vi "Process.vi"(8 "error in (no error)":errorcluster, 11 "Analyzer":refnum<class "Analyzer.lvclass">) -> (0 "error out":errorcluster, 3 "Analyzer out":refnum<class "Analyzer.lvclass">)   [LabVIEW 2022 SP3, in "Analyzer.lvclass"]
uses:
  Analyzer.lvclass
  C:/Program Files (x86)/National Instruments/LabVIEW 2022/vi.lib/JKI/JKI SMO/SMO/SMO.lvclass
  <vilib>/JKI/JKI SMO/SMO/Typedefs/Parent Call--Enum.ctl
  Typedefs/PublicEvents--Analyzer.NewEventMessage.ctl
  <vilib>/JKI/JKI SMO/SMO/SMO.lvclass
  <vilib>/JKI/JKI SMO/SMO/SMO.lvclass/SMO.ctl
  2a4e98fd-c6f0-4dfa-82c0-cf19db74dbf6.vi
  <vilib>/JKI/JKI SMO/SMO/Private/GetVariant(Attr).vi
  <vilib>/JKI/JKI SMO/Support/Attribute.Identity/Read UniqueName.vi
  <vilib>/JKI/JKI SMO/Support/Attribute.Identity/Read Given Name.vi
  <vilib>/JKI/JKI SMO/Support/Attribute.Identity/Read ProspectiveOwner.vi
  <vilib>/JKI/JKI SMO/SMO/Private/ReftoDVR--SMO.vi
  <vilib>/Utility/file.llb/Write Delimited Spreadsheet (string).vi
  <vilib>/JKI/JKI SMO/Support/Attribute.Identity/Attribute.Identity.lvclass
panel:
  in  "Save":bool
  in  "Word or Phrase:":string
  in  "Search By:":string(combo)
  in  "Start Button":bool
  out "Table Report":string[][](table)
  in  "OK":bool
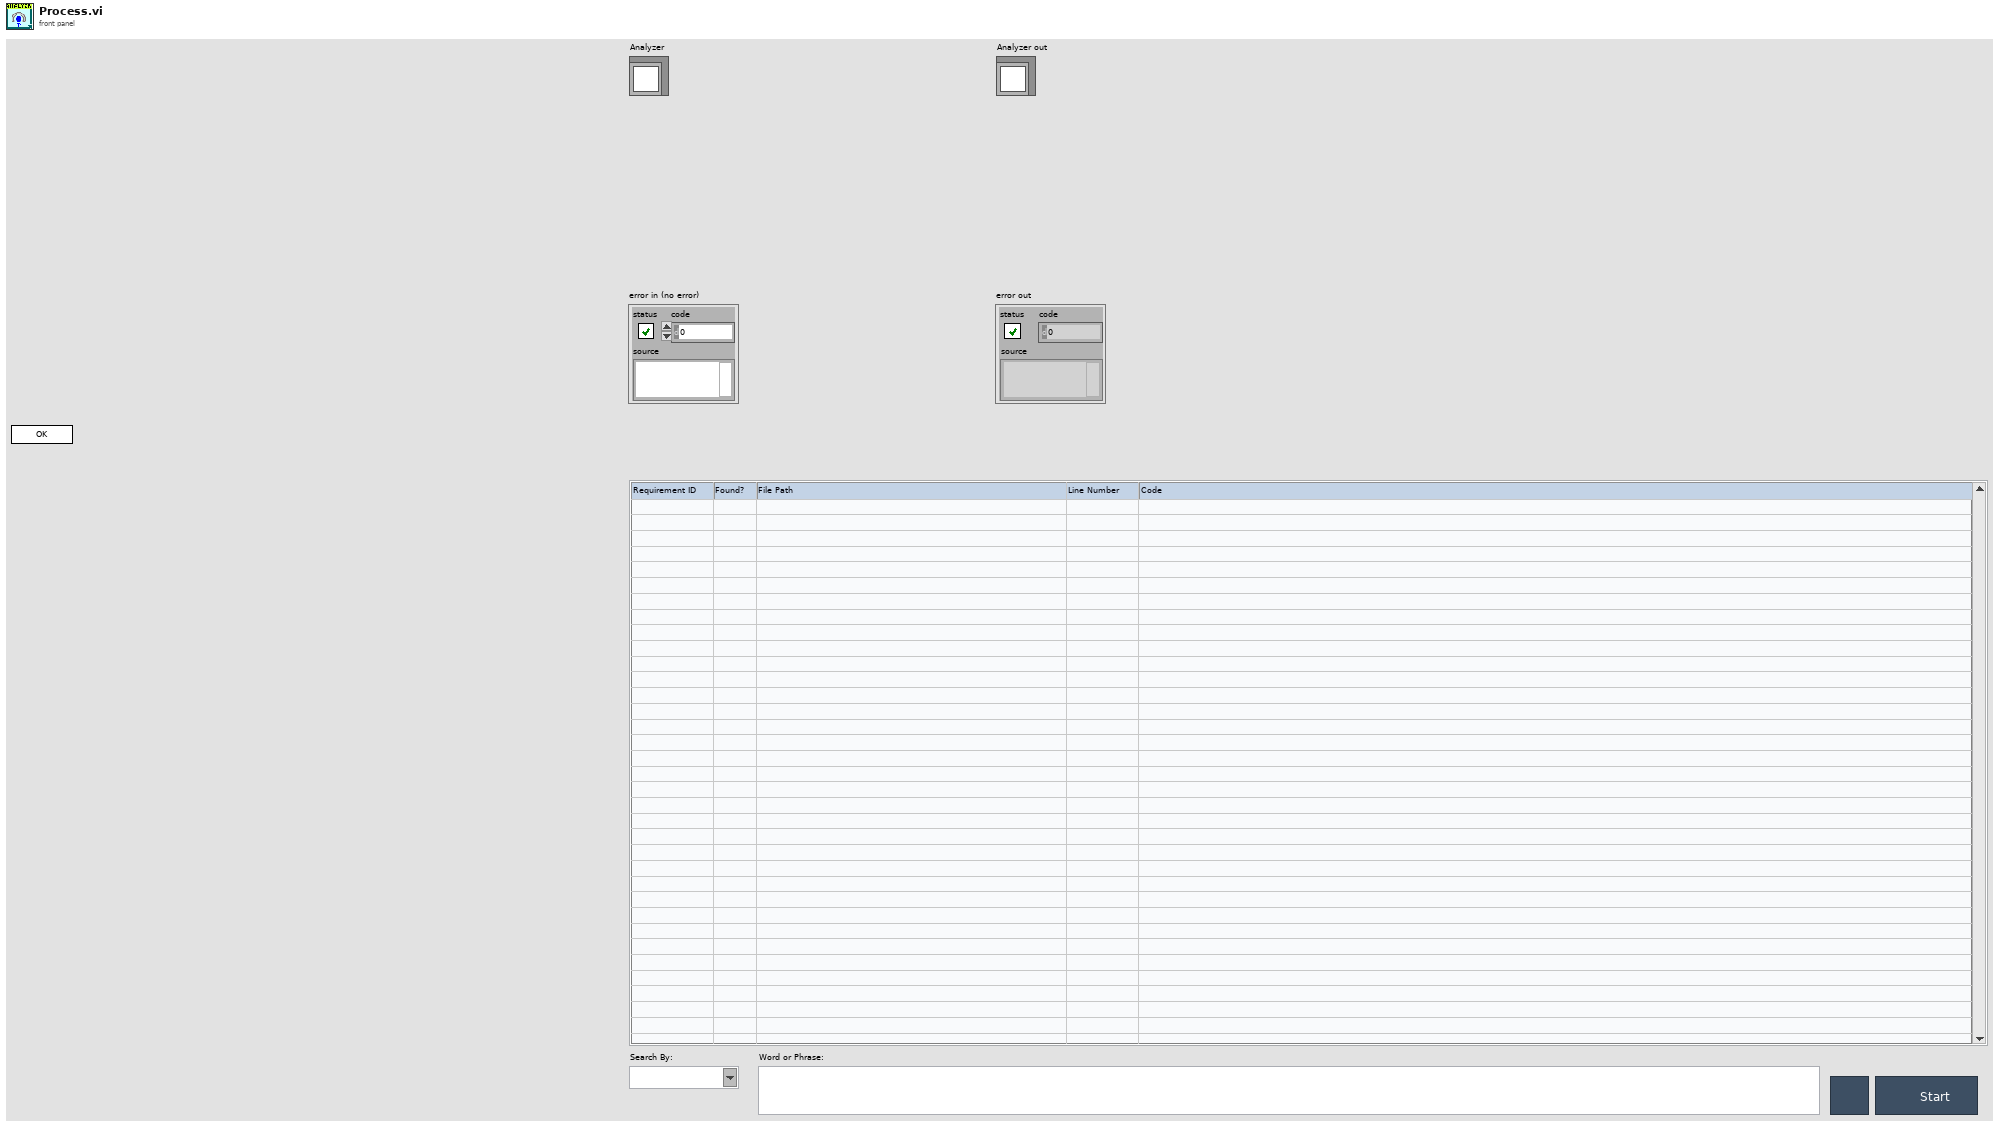
[diagram p1: front panel]
types:
  T1 = typedef "SMO.lvclass/Parent Call--Enum.ctl" = enum16{"Allows parent to run", "Does not request parent to run"}
  T2 = typedef "Analyzer.lvclass/PublicEvents--Analyzer.NewEventMessage.ctl" = cluster{"Title":string, "Message":variant}
  T3 = cluster{"Requirements Directory":path, "Report Generation Save Path":path, "Source Code to Directory":path, "Search By:":string, "Word/Phrase:":string, "Source Code File":path}
  T4 = enum8{"Enabled", "Disabled", "Disabled and Grayed Out"}
  T5 = enum32{"invalid app kind", "Development System", "Run Time System", "Student Edition", "Embedded LabVIEW", "Evaluation", "Custom"}
  T6 = enum32{"Invalid", "Standard", "Closed", "Hidden", "Minimized", "Maximized"}
  T7 = typedef "Analyzer.lvclass/Analyzer State--enum.ctl" = enum16{"unknown", "Opened", "Embedded", "Closed"}
  T8 = cluster{"Requirements Directory":path, "Report Generation Save Path":path, "Source Code Directory":path, "Search By:":string, "Word/Phrase:":string, "Source Code File":path}
  T9 = cluster{"Core":cluster{"Current VI Reference":refnum<vi>, "Close Panel on Exit?":bool, "error":errorcluster}, "Self Ref":refnum<class "Analyzer.lvclass">, "Python":cluster{"Ref":refnum<k35>, "SReTT_script":path}, "Settings":cluster{"Requirements Directory":path, "Report Generation Save Path":path, "Source Code Directory":path, "Search By:":string, "Word/Phrase:":string, "Source Code File":path}, "Table":string[][], "Requirement to Look":string, "Requirements":string[], "Req Files Done":bool, "Code Files Done":bool, "Single Word":bool, "S Word Ctrl":bool}
  T10 = cluster{"Current VI Reference":refnum<vi>, "Close Panel on Exit?":bool, "error":errorcluster}
  T11 = typedef "SMO.lvclass/Protected Events.ctl" = cluster{"StopProcesses":refnum<user-event>, "AbortProcesses":refnum<user-event>, "Config Changed":refnum<user-event>, "Dependency":refnum<user-event>}
  T12 = typedef "Analyzer.lvclass/PublicEvents--Cluster.ctl" = cluster{"UI State":refnum<user-event>, "NewEventMessage":refnum<user-event>}
  T13 = typedef "Analyzer.lvclass/PrivateEvents--Cluster.ctl" = cluster{"NewRequest":refnum<user-event>}
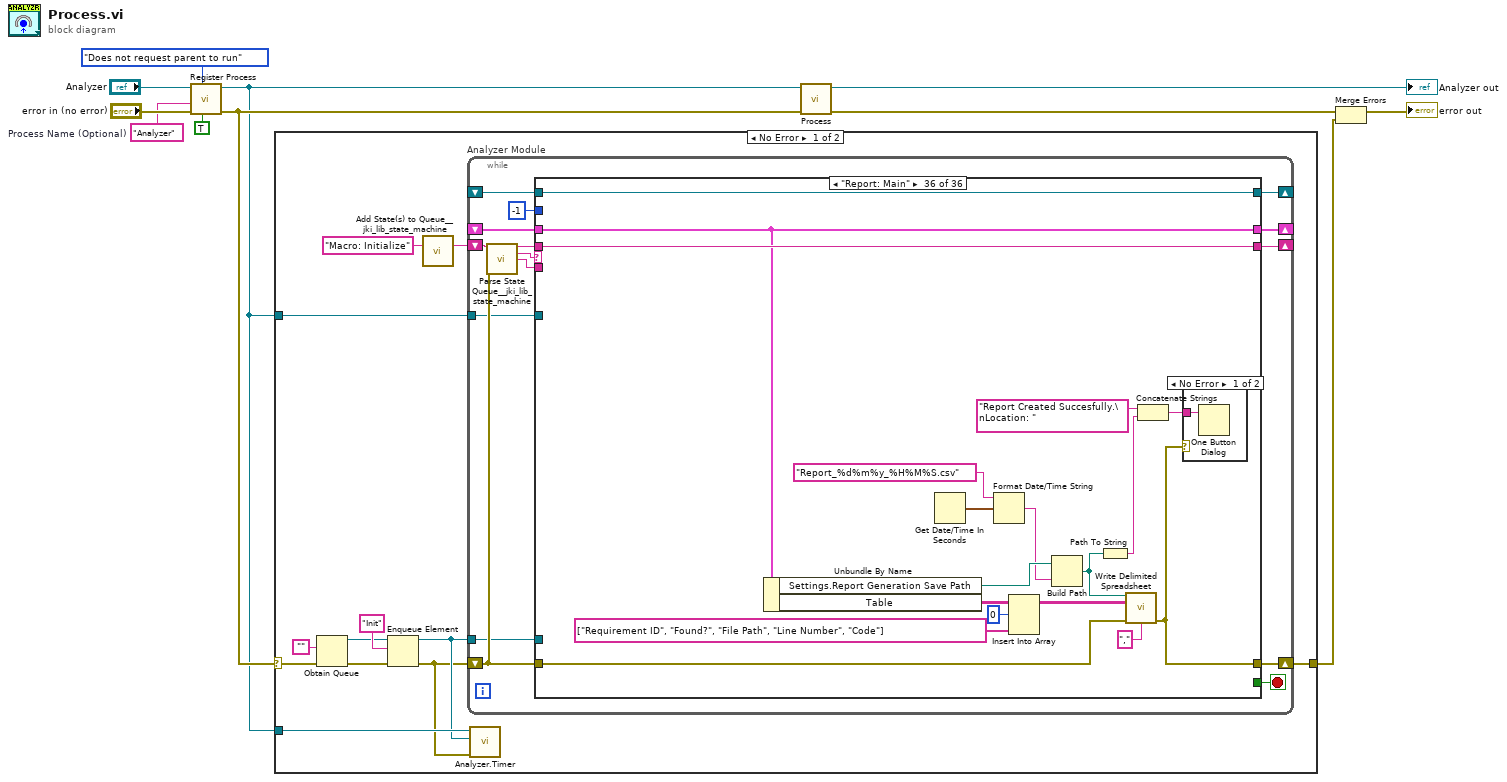
[diagram p0: block diagram]
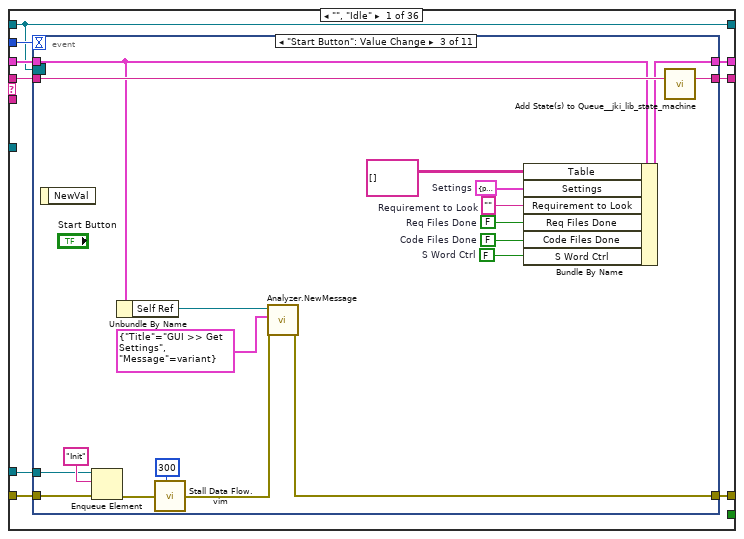
[diagram p2: hidden frame]
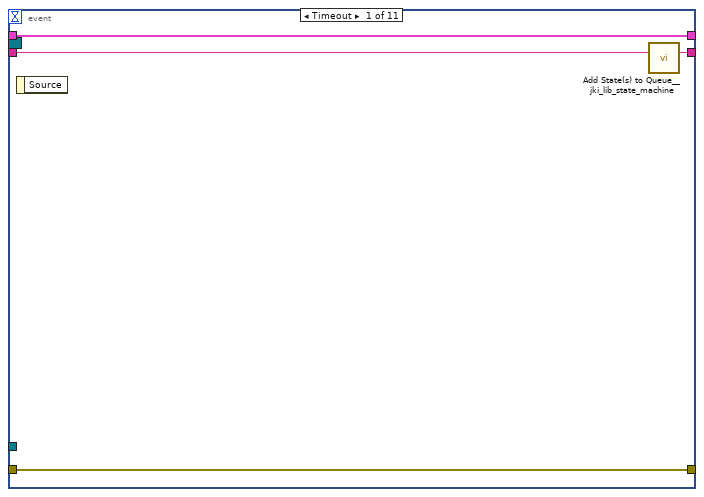
[diagram p3: hidden frame]
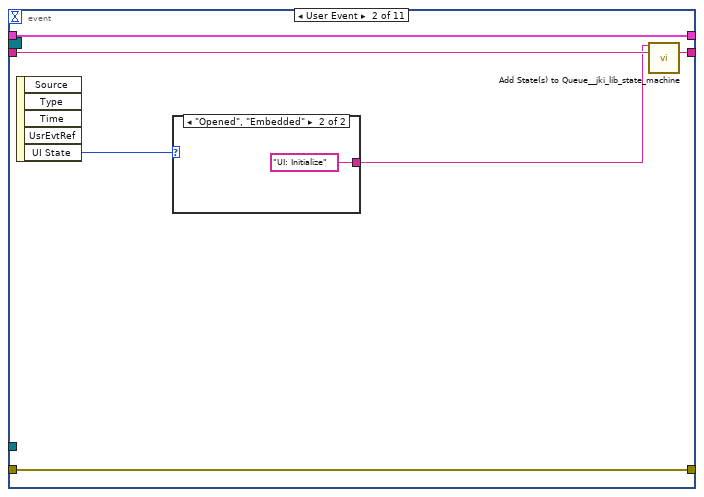
[diagram p4: hidden frame]
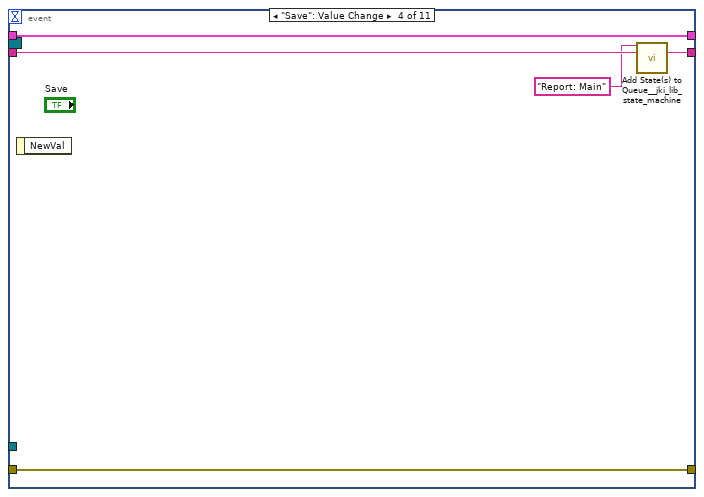
[diagram p6: hidden frame]
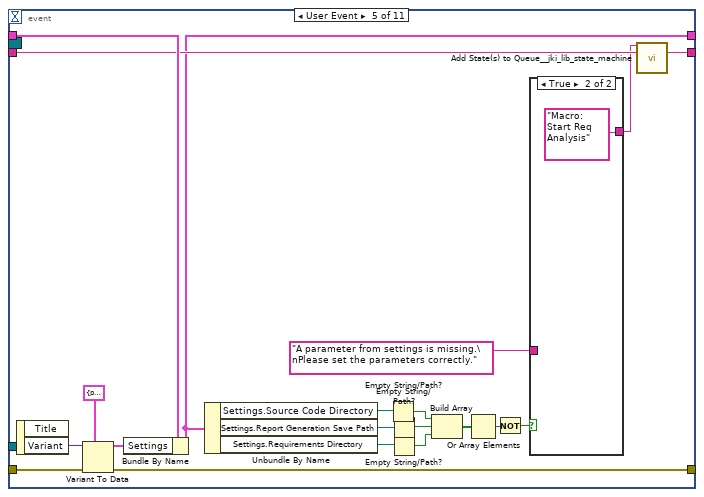
[diagram p7: hidden frame]
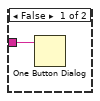
[diagram p8: hidden frame]
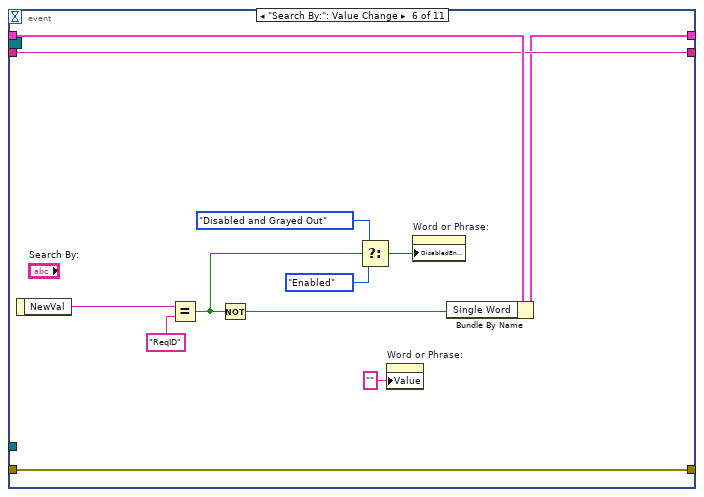
[diagram p9: hidden frame]
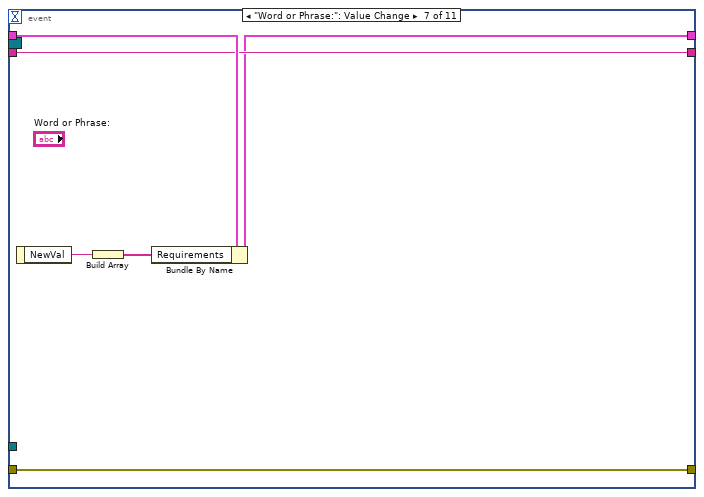
[diagram p10: hidden frame]
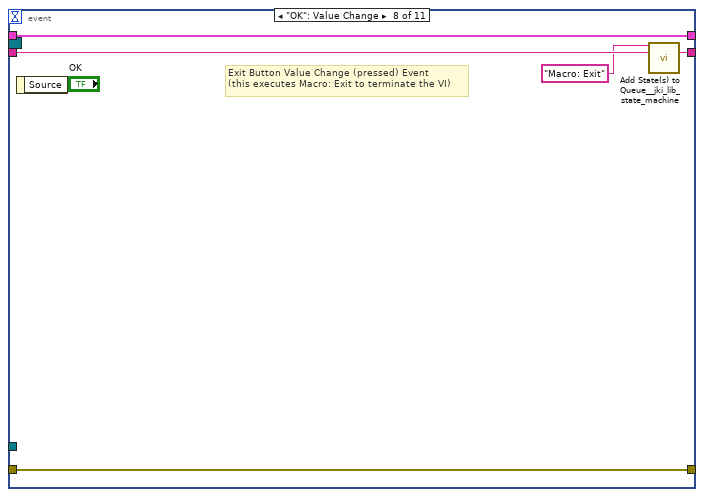
[diagram p11: hidden frame]
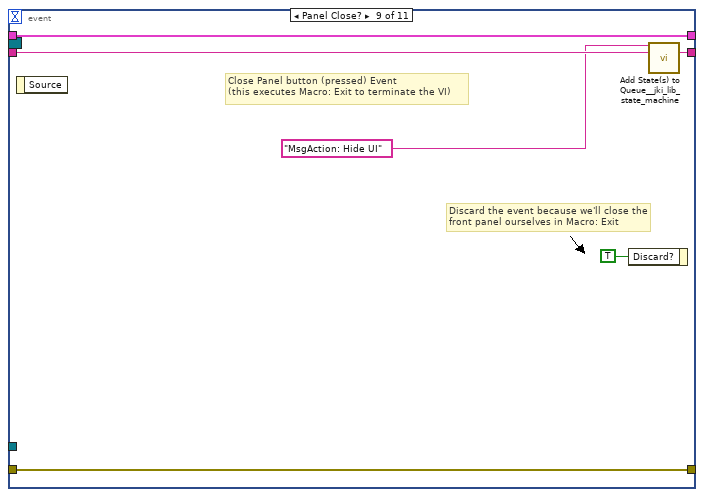
[diagram p12: hidden frame]
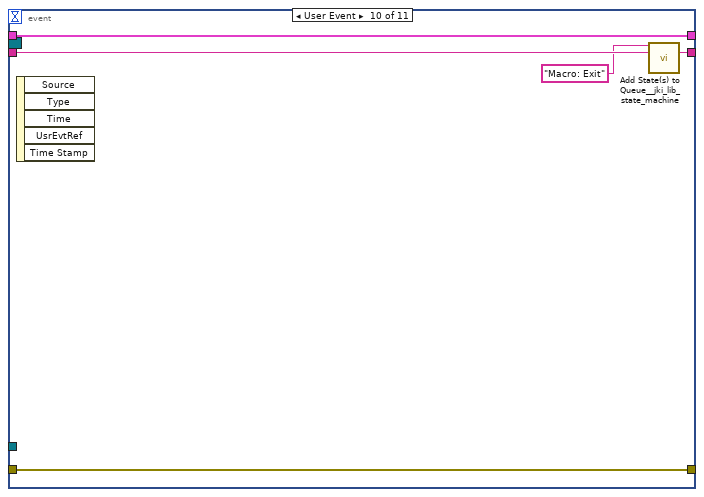
[diagram p13: hidden frame]
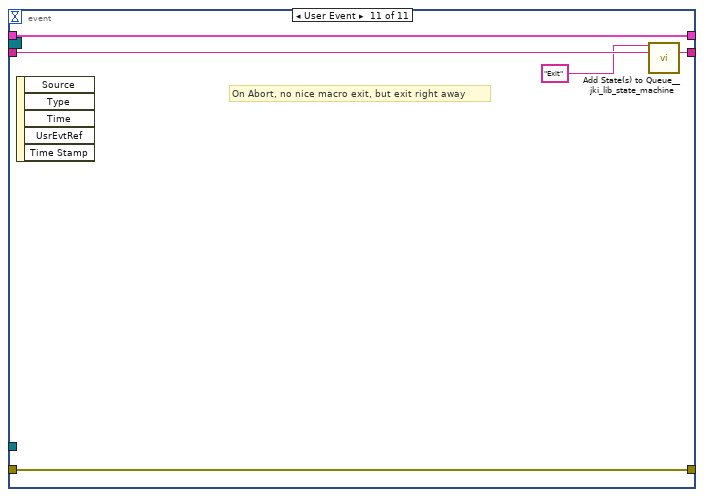
[diagram p14: hidden frame]
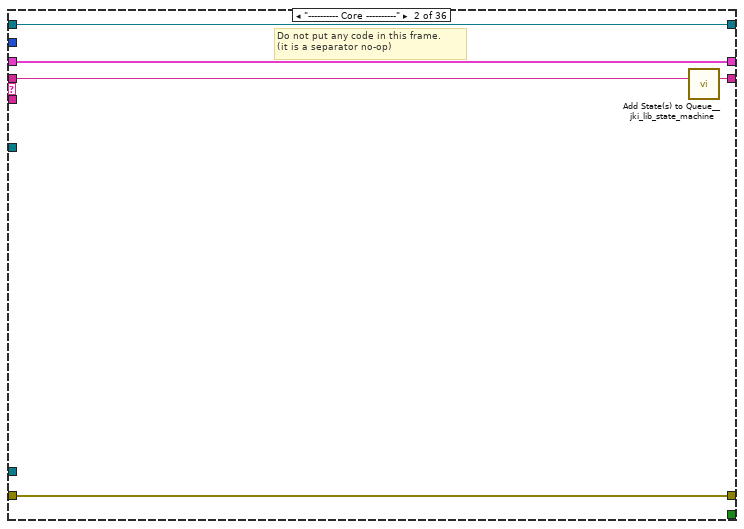
[diagram p15: hidden frame]
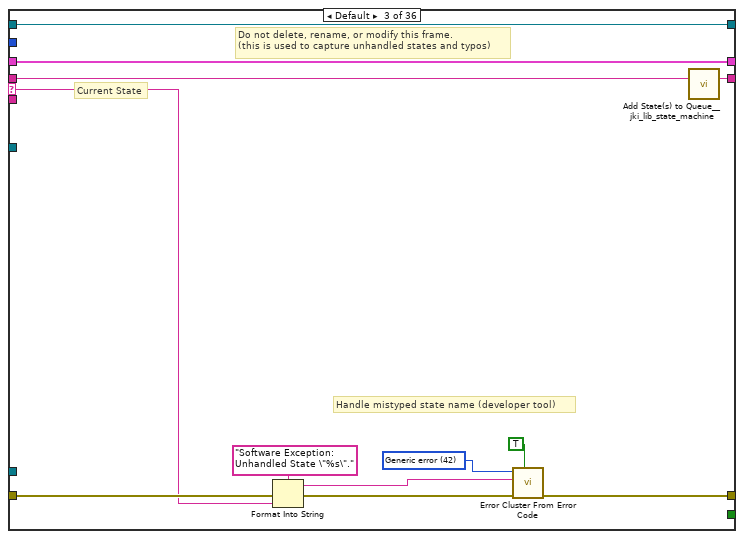
[diagram p16: hidden frame]
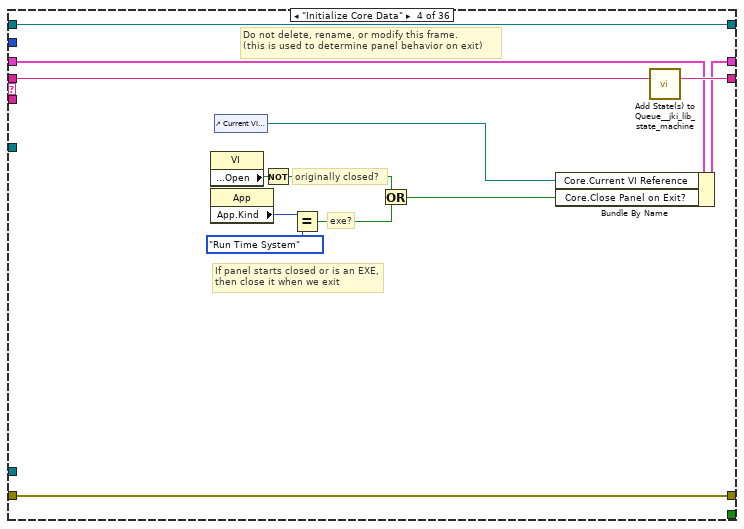
[diagram p17: hidden frame]
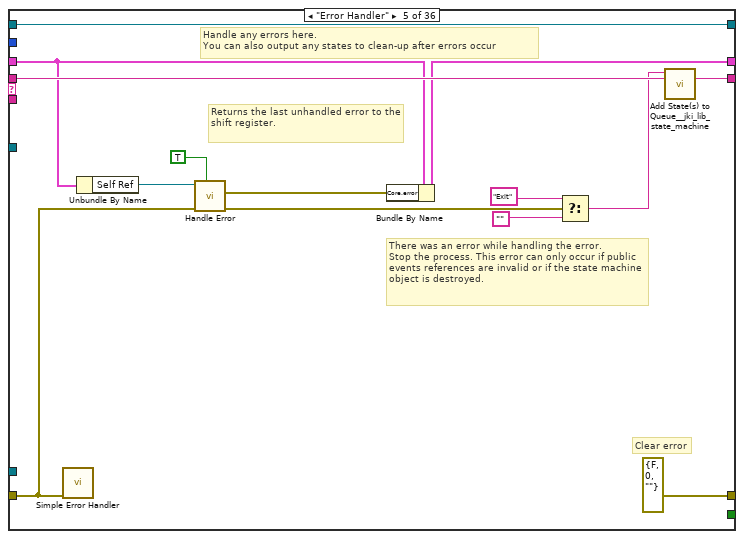
[diagram p18: hidden frame]
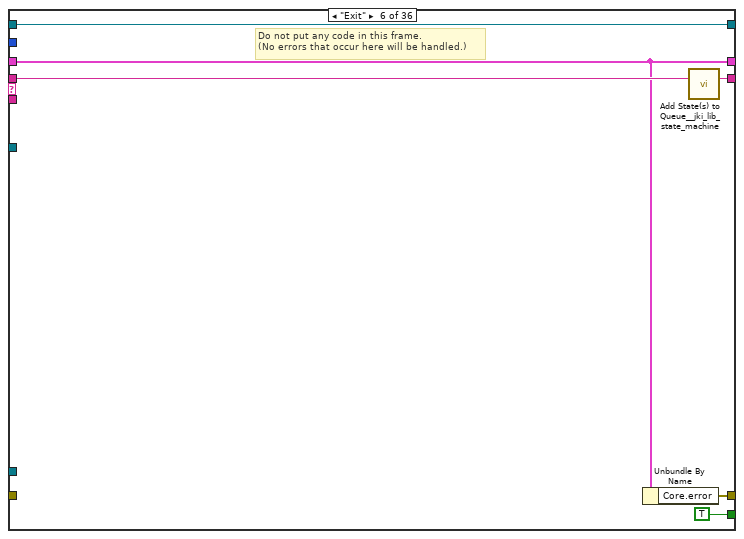
[diagram p19: hidden frame]
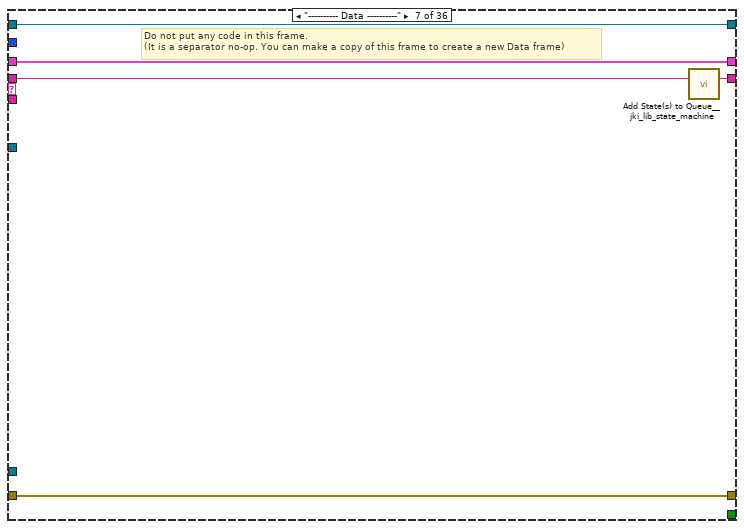
[diagram p20: hidden frame]
diagram:
  w5 = "Analyzer"  # Process Name (Optional)
  n1 = call <vilib>:"Register Process.vi"("Forces Self to Run (F)"=TRUE, "Parent Call"=Parent_Call--Enum."Does not request parent to run", "error in (no error)"="error in (no error)", "Process Name (optional)"=w5, "SMO"="Analyzer") -> ("error out"=w11:errorcluster, "SMO out"=w1:refnum<class "Analyzer.lvclass">)  [unwired: 5 in]
  n2 = case shown="No Error" w11 {
    selector: w11 -> [w19 w546]
    tunnel: w1 -> [w21 _]
    tunnel: [w20 w546] -> w9
    tunnel: w1 -> [w14 _]
    frame No Error {
      n3 = Obtain Queue(element data type="", error in (no error)=w19) -> (queue out=w16:refnum<queue>, error out=w15:errorcluster)  [unwired: 3 in, 1 out]
      n4 = Enqueue Element(queue=w16, element="Init", error in (no error)=w15) -> (queue out=w13:refnum<queue>, error out=w12:errorcluster)  [unwired: 1 in, 1 out]
      n5 = call <vilib>:"Add State(s) to Queue__jki_lib_state_machine.vi"("State(s) in (\"\")"="Macro: Initialize") -> ("States Out"=w23:string)  [unwired: 14 in]
      n6 = while "Analyzer Module" {
        shift-right: [w31] -> _
        shift-left: _ -> [w30]
        shift-right: [w34] -> w20
        shift-left: w12 -> [w28]
        shift-right: [w33] -> _
        shift-left: w23 -> [w35]
        tunnel: w21 -> [w27]
        shift-right: [w26] -> _
        shift-left: _ -> [w25]
        tunnel: w13 -> [w24]
        stop <- w32 stop-if-true
        n7 = call <vilib>:"Parse State Queue__jki_lib_state_machine.vi"("State Queue"=w35, "Error In (no error)"=w28) -> ("Remaining States"=w37:string, "Current State"=w38:string, "Arguments"=w36:string)  [unwired: 11 in]
        n8 = case shown="\"Report: Main\"" w38 {
          selector: w38 -> [_ _ w150 _ _ _ _ _ _ _ _ _ _ _ _ _ _ _ _ _ _ _ _ _ _ _ _ _ _ _ _ _ _ _ _ _]
          tunnel: w37 -> [w47 w148 w154 w173 w187 w193 w198 w226 w240 w245 w250 w256 w263 w279 w311 w320 w326 w337 w342 w353 w365 w370 w385 w391 w393 w408 w423 w440 w450 w469 w473 w481 w507 w520 w524 w543]
          tunnel: w36 -> [_ _ _ _ _ _ _ _ _ _ _ _ w257 w275 _ _ _ _ _ _ _ _ _ _ _ _ _ _ _ _ _ _ _ w516 _ _]
          tunnel: w30 -> [w45 w145 w152 w164 w183 w188 w195 _ w236 w242 w248 w253 w261 w277 w308 w317 w323 w328 w339 w350 w362 w367 w383 w389 w394 w405 w428 w441 w456 w470 w472 w484 w511 w521 w525 w542]
          tunnel: [w44 w146 w156 w170 errorcluster {"status"=FALSE, "code"=0, "source"=""} ("error out") w189 w196 w199 w237 w243 w247 w252 w258 w272 w309 w312 w324 w335 w340 w344 w360 w368 w381 w387 w392 w402 w427 w439 w455 w468 w475 w486 w505 w517 w523 w531] -> w34
          tunnel: w28 -> [w43 w146 w155 w170 w174 _ w196 w209 w230 w243 w247 w252 w259 w273 w309 w312 w324 w335 w340 w345 w357 w368 w375 w387 w392 w406 w415 w439 w457 w468 w475 w486 w506 w518 w523 w540]
          tunnel: [w46 w147 w153 w172 w186 w192 w197 w225 w239 w244 w249 w255 w262 w278 w310 w319 w325 w336 w341 w352 w364 w369 w384 w390 w393 w408 w424 w440 w451 w469 w474 w482 w508 w520 w524 w543] -> w33
          tunnel: [_ _ _ _ _ TRUE _ _ _ _ _ _ _ _ _ _ _ _ _ _ _ _ _ _ _ _ _ _ _ _ _ _ _ _ _ _] -> w32
          tunnel: [w42 w145 w152 w171 w182 w188 w195 w224 w236 w242 w248 w253 w261 w277 w308 w317 w323 w328 w339 w350 w362 w367 w383 w389 w394 w403 w421 w441 w443 w470 w472 w479 w510 w521 w525 w542] -> w31
          tunnel: -1 ("Timeout") -> [w41 _ _ _ _ _ _ _ _ _ _ _ _ _ _ _ _ _ _ _ _ _ _ _ _ _ _ _ _ _ _ _ _ _ _ _]
          tunnel: w27 -> [_ _ _ _ _ _ _ w223 _ _ _ _ _ _ _ _ _ _ _ _ _ _ _ _ _ _ _ _ _ _ _ _ _ _ _ _]
          tunnel: [w40 w144 w149 w161 w185 w190 w194 w222 w235 w241 w246 w254 w260 w276 w307 w318 w322 w329 w338 w351 w363 w366 w380 w388 w395 w409 w429 w442 w458 w471 w476 w487 w515 w522 w526 w544] -> w26
          tunnel: w25 -> [w40 w144 w149 w161 w185 w190 w194 w222 w235 w241 w246 w254 w260 w276 w307 w318 w322 w329 w338 w351 w363 w366 _ w388 w395 w409 w429 w442 w458 w471 w476 w487 w515 w522 w526 w544]
          tunnel: w24 -> [w39 _ _ _ _ _ _ _ w232 _ _ _ _ _ _ _ _ _ _ _ _ _ _ _ _ _ _ _ _ _ _ _ _ w519 _ _]
          frame "", "Idle" {
            n9 = event shown="[2] \"Start Button\": Value Change" {
              selector: w40 -> [_ _ _ _ _ _ _ _ _ _ _]
              dyn-events: _ -> [_ _ _ _ _ _ _ _ _ _ _]
              timeout: w41 -> [_ _ _ _ _ _ _ _ _ _ _]
              tunnel: w47 -> [w51 w57 w76 w79 w97 w115 w121 w127 w133 w138 w143]
              tunnel: [w50 w56 w77 w80 w98 w115 w121 w126 w132 w137 w142] -> w46
              tunnel: w45 -> [w48 w54 w75 w82 w102 w116 w122 w124 w129 w135 w140]
              tunnel: [w49 w55 w73 w81 w99 w114 w120 w125 w131 w136 w141] -> w44
              tunnel: w43 -> [w49 w55 w63 w81 w100 w114 w120 w125 w131 w136 w141]
              tunnel: [w48 w54 w71 w82 w96 w109 w119 w124 w129 w135 w140] -> w42
              tunnel: w39 -> [_ _ w64 _ _ _ _ _ _ _ _]
              event Timeout {
                n10 = event-data() -> ()  [unwired: 1 in, 1 out]
                n11 = call <vilib>:"Add State(s) to Queue__jki_lib_state_machine.vi"("State(s) in (\"\")"=w51) -> ("States Out"=w50:string)  [unwired: 14 in]
              }
              event User Event {
                n12 = event-data() -> ("UI State"=w53:T7)  [unwired: 1 in, 4 out]
                n13 = case shown="\"Opened\", \"Embedded\"" w53 {
                  tunnel: [_ "UI: Initialize" ("State(s) in Front (\"\")")] -> w52
                  frame Default {
                  }
                  frame "Opened", "Embedded" {
                  }
                }
                n14 = call <vilib>:"Add State(s) to Queue__jki_lib_state_machine.vi"("State(s) in Front (\"\")"=w52, "State(s) in (\"\")"=w57) -> ("States Out"=w56:string)  [unwired: 13 in]
              }
              event "Start Button": Value Change {
                w66 = FALSE  # S Word Ctrl
                w67 = FALSE  # Code Files Done
                w68 = FALSE  # Req Files Done
                w69 = ""  # Requirement to Look
                w70 = T8 {"Requirements Directory"=path "", "Report Generation Save Path"=path "", "Source Code Directory"=path "", "Search By:"="", "Word/Phrase:"="", "Source Code File"=path ""}  # Settings
                n15 = event-data() -> ()  [unwired: 1 in, 1 out]
                n16 = Enqueue Element(queue=w64, element="Init", error in (no error)=w63) -> (error out=w62:errorcluster)  [unwired: 1 in, 2 out]
                n17 = Unbundle By Name(w75) -> ("Self Ref"=w74:refnum<class "Analyzer.lvclass">)
                n18 = call "Stall Data Flow.vim"("value in"=w62, "milliseconds to wait"=u32 300) -> ("value out"=w60:errorcluster)  [unwired: 1 out]
                n19 = call "Analyzer.NewMessage.vi"("error in (no error)"=w60, "event data"=T2 {"Title"="GUI >> Get Settings", "Message"=variant}, "Analyzer in"=w74) -> ("error out"=w73:errorcluster)  [unwired: 7 in, 1 out]
                n20 = Bundle By Name(cluster=w75, "Table"=string[][] [], "Settings"=w70, "Requirement to Look"=w69, "Req Files Done"=w68, "Code Files Done"=w67, "S Word Ctrl"=w66) -> (w71:T9)
                n21 = call <vilib>:"Add State(s) to Queue__jki_lib_state_machine.vi"("State(s) in (\"\")"=w76) -> ("States Out"=w77:string)  [unwired: 14 in]
              }
              event "Save": Value Change {
                n22 = event-data() -> ()  [unwired: 1 in, 1 out]
                n23 = call <vilib>:"Add State(s) to Queue__jki_lib_state_machine.vi"("State(s) in Front (\"\")"="Report: Main" ("State(s) in Front (\"\")"), "State(s) in (\"\")"=w79) -> ("States Out"=w80:string)  [unwired: 13 in]
              }
              event User Event {
                n24 = event-data() -> ("Variant"=w101:variant)  [unwired: 1 in, 1 out]
                n25 = Variant To Data(error in=w100, type=T3 {"Requirements Directory"=path "", "Report Generation Save Path"=path "", "Source Code to Directory"=path "", "Search By:"="", "Word/Phrase:"="", "Source Code File"=path ""} ("New Settings Config 2"), Variant=w101) -> (data=w84:T3, error out=w99:errorcluster)
                n26 = Bundle By Name(cluster=w102, "Settings"=w84) -> (w96:T9)
                n27 = Unbundle By Name(w96) -> ("Settings.Source Code Directory"=w95:path, "Settings.Report Generation Save Path"=w94:path, "Settings.Requirements Directory"=w93:path)
                n28 = Empty String/Path?(string/path=w95) -> (empty?=w91:bool)
                n29 = Empty String/Path?(string/path=w94) -> (empty?=w92:bool)
                n30 = Empty String/Path?(string/path=w93) -> (empty?=w90:bool)
                n31 = Build Array(w91, w92, w90) -> (w89:bool[])
                n32 = Or Array Elements(Boolean array=w89) -> (logical OR=w88:bool)
                n33 = Not(x=w88) -> (.not. x?=w87:bool)
                n34 = case shown="True" w87 {
                  tunnel: "A parameter from settings is missing.\nPlease set the parameters correctly." -> [w103 _]
                  tunnel: [_ "Macro: Start Req Analysis"] -> w85
                  frame False {
                    n35 = One Button Dialog(message=w103) -> ()  [unwired: 1 in, 1 out]
                  }
                  frame True {
                  }
                }
                n36 = call <vilib>:"Add State(s) to Queue__jki_lib_state_machine.vi"("State(s) in Front (\"\")"=w85, "State(s) in (\"\")"=w97) -> ("States Out"=w98:string)  [unwired: 13 in]
              }
              event "Search By:": Value Change {
                n37 = event-data() -> ("NewVal"=w107:string)  [unwired: 1 in]
                n38 = Equal?(x=w107, y="ReqID") -> (x = y?=w106:bool)
                n39 = Not(x=w106) -> (.not. x?=w108:bool)
                n40 = Select(t=T4."Disabled and Grayed Out" ("Disabled"), s=w106, f=T4."Enabled") -> (s? t:f=w111:T4)
                n41 = property on="Word or Phrase:" class="Str"("Value"="" ("Word or Phrase:")) -> ()  [unwired: 2 in, 2 out]
                n42 = property on="Word or Phrase:" class="Str"("DisabledEnum"=w111) -> ()  [unwired: 2 in, 2 out]
                n43 = Bundle By Name(cluster=w116, "Single Word"=w108) -> (w109:T9)
              }
              event "Word or Phrase:": Value Change {
                n44 = event-data() -> ("NewVal"=w118:string)  [unwired: 1 in]
                n45 = Build Array(w118) -> (w117:string[])
                n46 = Bundle By Name(cluster=w122, "Requirements"=w117) -> (w119:T9)
              }
              event "OK": Value Change {
                # "Exit Button Value Change (pressed) Event\n(this executes Macro: Exit to terminate the VI)"
                n47 = event-data() -> ()  [unwired: 1 in, 1 out]
                n48 = call <vilib>:"Add State(s) to Queue__jki_lib_state_machine.vi"("State(s) in Front (\"\")"="Macro: Exit", "State(s) in (\"\")"=w127) -> ("States Out"=w126:string)  [unwired: 13 in]
              }
              event Panel Close? {
                # "Discard the event because we'll close the front panel ourselves in Macro: Exit"
                # "Close Panel button (pressed) Event\n(this executes Macro: Exit to terminate the VI)"
                n49 = event-data() -> ()  [unwired: 1 in, 1 out]
                n50 = event-data("Discard?"=TRUE) -> ()  [unwired: 1 in, 1 out]
                n51 = call <vilib>:"Add State(s) to Queue__jki_lib_state_machine.vi"("State(s) in Front (\"\")"="MsgAction: Hide UI", "State(s) in (\"\")"=w133) -> ("States Out"=w132:string)  [unwired: 13 in]
              }
              event User Event {
                n52 = event-data() -> ()  [unwired: 1 in, 5 out]
                n53 = call <vilib>:"Add State(s) to Queue__jki_lib_state_machine.vi"("State(s) in Front (\"\")"="Macro: Exit", "State(s) in (\"\")"=w138) -> ("States Out"=w137:string)  [unwired: 13 in]
              }
              event User Event {
                # "On Abort, no nice macro exit, but exit right away"
                n54 = event-data() -> ()  [unwired: 1 in, 5 out]
                n55 = call <vilib>:"Add State(s) to Queue__jki_lib_state_machine.vi"("State(s) in Front (\"\")"="Exit", "State(s) in (\"\")"=w143) -> ("States Out"=w142:string)  [unwired: 13 in]
              }
            }
          }
          frame "---------- Core ----------" {
            # "Do not put any code in this frame.\n(it is a separator no-op)"
            n56 = call <vilib>:"Add State(s) to Queue__jki_lib_state_machine.vi"("State(s) in (\"\")"=w148) -> ("States Out"=w147:string)  [unwired: 14 in]
          }
          frame Default {
            w159 = 42 items=["No error", "Argument error", "Memory is full", "Out of zone", "End of file", "File already open", "Generic file I/O error", "File not found", "File permission error", "Disk is full", "Duplicate path", "Too many files open", "System feature not enabled", "Resource file not found", "Cannot add resource", "Resource not found", "Image not found", "Image memory error", "Pen does not exist", "Config type invalid", "Config token not found", "Config parse error", "Config memory error", "Bad external code format", "Bad external code offset", "External code not present", "Null window", "Destroy window error", "Null menu", "Print aborted", "Bad print record", "Print driver error", "Windows error during printing", "Memory error during printing", "Print dialog error", "Generic print error", "Invalid device refnum", "Device not found", "Device parameter error", "Device unit error", "Cannot open device", "Device call aborted", "Generic error", "Cancelled by user", "Object ID too low", "Object ID too high", "Object not in heap", "Unknown heap", "Unknown object (invalid DefProc)", "Unknown object (DefProc not in table)", "Message out of range", "Invalid (null) method", "Unknown message", "Manager call not supported", "Bad address", "Network operation in progress", "Network operation timed out", "Connection is busy", "Network attribute not supported", "Network error", "Address in use", "System out of memory", "Connection aborted", "Connection refused", "Not connected", "Already connected", "Connection closed", "Initialization error (interapplication manager)", "Bad occurrence", "Wait on unbound occurrence handler", "Occurrence queue overflow", "Datalog type conflict", "Unused", "Unrecognized type (interapplication manager)", "Memory corrupt", "Failed to make temporary DLL", "Old CIN version", "Drag socket not found", "Failed to load drop-object", "Failed to register OLE object", "Failed to release OLE object", "Format specifier type mismatch", "Unknown format specifier", "Too few format specifiers", "Too many format specifiers", "Scan failed", "Newer CIN version", "Error converting to variant", "Runtime menu error", "Password tampered", "Variant attribute not found", "Incompatible variant data type", "Event data is not available", "Event Store is not present", "Occurrence is not found", "Event Queue is not created", "Event info is not available", "Refnum passed is NULL", "Error retrieving Class GUID", "Error retrieving CoClass GUID", "Error retrieving TypeLib GUID.", "Bad built application magic bytes.", "Specific driver is different from the specific driver associated with the Logical Name.", "There is no session opened to the class driver.", "Max Error", "MAX - Error with config objects", "MAX - Error loading configuration", "MAX - Group not supported"]
            # "Current State"
            # "Do not delete, rename, or modify this frame.\n(this is used to capture unhandled states and typos)"
            # "Handle mistyped state name (developer tool)"
            n57 = Format Into String(format string="Software Exception: Unhandled State \"%s\"." ("message"), error in=w155, w150) -> (resulting string=w158:string, error out=w157:errorcluster)  [unwired: 1 in]
            n58 = call <vilib>:"Error Cluster From Error Code.vi"("show call chain? (False)"=TRUE, "error in (no error)"=w157, "error message (\"\")"=w158, "error code (0)"=w159) -> ("error out"=w156:errorcluster)  [unwired: 5 in]
            n59 = call <vilib>:"Add State(s) to Queue__jki_lib_state_machine.vi"("State(s) in (\"\")"=w154) -> ("States Out"=w153:string)  [unwired: 14 in]
          }
          frame "Initialize Core Data" {
            # "Do not delete, rename, or modify this frame.\n(this is used to determine panel behavior on exit)"
            # "originally closed?"
            # "exe?"
            # "If panel starts closed or is an EXE, then close it when we exit"
            n60 = property class="VI"() -> ("Front Panel.Open"=w169:bool)  [unwired: 2 in, 2 out]
            n61 = property class="App"() -> ("App.Kind"=w168:T5)  [unwired: 2 in, 2 out]
            n62 = control-ref of="Current VI Reference"() -> (w162:refnum<vi>)
            n63 = Not(x=w169) -> (.not. x?=w166:bool)
            n64 = Equal?(x=w168, y=T5."Run Time System" ("Application:Kind")) -> (x = y?=w165:bool)
            n65 = Or(x=w166, y=w165) -> (x .or. y?=w163:bool)
            n66 = Bundle By Name(cluster=w164, "Core.Current VI Reference"=w162, "Core.Close Panel on Exit?"=w163) -> (w171:T9)
            n67 = call <vilib>:"Add State(s) to Queue__jki_lib_state_machine.vi"("State(s) in (\"\")"=w173) -> ("States Out"=w172:string)  [unwired: 14 in]
          }
          frame "Error Handler" {
            # "Returns the last unhandled error to the shift register."
            # "There was an error while handling the error.\nStop the process. This error can only occur if public events references are invalid or if the state machine object is destroyed."
            # "Handle any errors here.\nYou can also output any states to clean-up after errors occur"
            # "Clear error"
            n68 = call <vilib>:"Simple Error Handler.vi"("error in (no error)"=w174) -> ()  [unwired: 4 in, 5 out]
            n69 = Unbundle By Name(w183) -> ("Self Ref"=w184:refnum<class "Analyzer.lvclass">)
            n70 = call-dynamic "Handle Error.vi"("Stop on Unhandled Error (T)"=TRUE, "error in"=w174, "SMO"=w184) -> ("handling error"=w179:errorcluster, "Unhandled error"=w181:errorcluster)  [unwired: 6 in, 1 out]
            n71 = Bundle By Name(cluster=w183, "Core.error"=w181) -> (w182:T9)
            n72 = Select(t="Exit", s=w179, f="") -> (s? t:f=w176:string)
            n73 = call <vilib>:"Add State(s) to Queue__jki_lib_state_machine.vi"("State(s) in Front (\"\")"=w176, "State(s) in (\"\")"=w187) -> ("States Out"=w186:string)  [unwired: 13 in]
          }
          frame "Exit" {
            # "Do not put any code in this frame.\n(No errors that occur here will be handled.)"
            n74 = Unbundle By Name(w188) -> ("Core.error"=w189:errorcluster)
            n75 = call <vilib>:"Add State(s) to Queue__jki_lib_state_machine.vi"("State(s) in (\"\")"=w193) -> ("States Out"=w192:string)  [unwired: 14 in]
          }
          frame "---------- Data ----------" {
            # "Do not put any code in this frame.\n(It is a separator no-op. You can make a copy of this frame to create a new Data frame)"
            n76 = call <vilib>:"Add State(s) to Queue__jki_lib_state_machine.vi"("State(s) in (\"\")"=w198) -> ("States Out"=w197:string)  [unwired: 14 in]
          }
          frame "Data: Initialize" {
            w201 = FALSE  # S Word Ctrl
            w202 = FALSE  # Single Word
            w203 = FALSE  # Code Files Done
            w204 = FALSE  # Req Files Done
            w206 = string[] []  # Requirements
            w208 = ""  # Requirement to Look
            w212 = string[][] []  # Table
            w213 = T8 {"Requirements Directory"=path "", "Report Generation Save Path"=path "", "Source Code Directory"=path "", "Search By:"="", "Word/Phrase:"="", "Source Code File"=path ""}  # Settings
            w216 = cluster{"Ref":refnum<k35>, "SReTT_script":path} {"Ref"=refnum, "SReTT_script"=path ""}  # Python
            w219 = T10 {"Current VI Reference"=refnum, "Close Panel on Exit?"=FALSE, "error"={"status"=FALSE, "code"=0, "source"=""}}  # Core
            w221 = refnum<class "Analyzer.lvclass"> refnum  # Self Ref
            # "do not delete - used by framework"
            # "Initialize the shift-register data, here.\n(data names are defined by what you wire into the bundle function)"
            n77 = Variant To Data(error in=w209, type=w221, Variant=w223) -> (data=w220:refnum<class "Analyzer.lvclass">, error out=w217:errorcluster)
            n78 = Open Python Session(python version="3.9" ("Python version"), 3:w217) -> (session out=w215:refnum<k35>, error out=w199:errorcluster)  [unwired: 1 in]
            n79 = disable-structure shown="RUN_TIME_ENGINE==True" {
              disable-tunnel: [path "Dependencies/SReTT.py" ("name or relative path") path "../001_Python/SReTT/SReTT.py" ("name or relative path")] -> w200
              frame condition #0 {
              }
              frame condition #1 (active) {
              }
            }
            n80 = call <vilib>:"Application Directory.vi"() -> ("Application Directory"=w211:path)
            n81 = Build Path(base path=w211, name or relative path=w200) -> (appended path=w210:path)
            n82 = property on="Word or Phrase:" class="Str"("DisabledEnum"=T4."Disabled and Grayed Out" ("Disabled")) -> ()  [unwired: 2 in, 2 out]
            n83 = Bundle(cluster=w216, "Ref"=w215, "SReTT_script"=w210) -> (w214:cluster{"Ref":refnum<k35>, "SReTT_script":path})
            n84 = property on="Table Report" class="Tbl (strict)"("Value"=string[][] [] ("Table Report")) -> ()  [unwired: 2 in, 2 out]
            n85 = call <vilib>:"Add State(s) to Queue__jki_lib_state_machine.vi"("State(s) in (\"\")"=w226) -> ("States Out"=w225:string)  [unwired: 14 in]
            n86 = Bundle("Core"=w219, "Self Ref"=w220, "Python"=w214, "Settings"=w213, "Table"=w212, "Requirement to Look"=w208, "Requirements"=w206, "Req Files Done"=w204, "Code Files Done"=w203, "Single Word"=w202, "S Word Ctrl"=w201) -> (w224:T9)  [unwired: 1 in]
          }
          frame "Data: Cleanup" {
            # "Cleanup any data and references, here.\n(this is called automatically, by the Macro: Exit)"
            n87 = Unbundle By Name(w236) -> ("Core.Current VI Reference"=w238:refnum<vi>, "Python.Ref"=w234:refnum<k35>)
            n88 = Enqueue Element(queue=w232, element="STOP", error in (no error)=w230) -> (error out=w229:errorcluster)  [unwired: 1 in, 2 out]
            n89 = Close Python Session(session in=w234, error in=w229) -> (11:w233:errorcluster)
            n90 = Close Reference(reference=w238, error in (no error)=w233) -> (error out=w237:errorcluster)
            n91 = call <vilib>:"Add State(s) to Queue__jki_lib_state_machine.vi"("State(s) in (\"\")"=w240) -> ("States Out"=w239:string)  [unwired: 14 in]
          }
          frame "---------- UI ----------" {
            # "Do not put any code in this frame.\n(It is a separator no-op. You can make a copy of this frame to create a new UI frame)"
            n92 = call <vilib>:"Add State(s) to Queue__jki_lib_state_machine.vi"("State(s) in (\"\")"=w245) -> ("States Out"=w244:string)  [unwired: 14 in]
          }
          frame "UI: Initialize" {
            n93 = call <vilib>:"Add State(s) to Queue__jki_lib_state_machine.vi"("State(s) in (\"\")"=w250) -> ("States Out"=w249:string)  [unwired: 14 in]
          }
          frame "UI: Update" {
            # "Do not put any code in this frame.\n(It is a separator no-op. You can make a copy of this frame to create a new UI frame)"
            n94 = Unbundle By Name(w253) -> ("Table"=→"Table Report":string[][])
            n95 = call <vilib>:"Add State(s) to Queue__jki_lib_state_machine.vi"("State(s) in (\"\")"=w256) -> ("States Out"=w255:string)  [unwired: 14 in]
          }
          frame "UI: Cursor Set" {
            # "Argument"
            # "Initialize the User Interface, here.\n(this is called automatically, by the Macro: Init)"
            n96 = disable-structure shown="Default" {
              disable-tunnel: w259 -> [w264 w267]
              disable-tunnel: [w264 w266] -> w258
              disable-tunnel: w257 -> [_ w265]
              frame condition #0 {
              }
              frame condition #1 (active) {
                n97 = case shown="\"Idle\", Default" w265 {
                  tunnel: w267 -> [w269 w271]
                  tunnel: [w268 w270] -> w266
                  frame "Idle", Default {
                    n98 = call <vilib>:"Unset Busy.vi"("error in (no error)"=w269) -> ("error out"=w268:errorcluster)  [unwired: 10 in]
                  }
                  frame "Busy" {
                    n99 = call <vilib>:"Set Busy.vi"("error in (no error)"=w271) -> ("error out"=w270:errorcluster)  [unwired: 9 in, 1 out]
                  }
                }
              }
            }
            n100 = call <vilib>:"Add State(s) to Queue__jki_lib_state_machine.vi"("State(s) in (\"\")"=w263) -> ("States Out"=w262:string)  [unwired: 14 in]
          }
          frame "UI: Front Panel State" {
            # "Argument"
            # "Set Front Panel Open or Closed\n(Usage: \"UI: Front Panel State >> Open|Close\")"
            n101 = Unbundle By Name(w277) -> ("Core.Current VI Reference"=w274:refnum<vi>)
            n102 = disable-structure shown="Default" {
              disable-tunnel: w273 -> [w283 w306]
              disable-tunnel: [w282 w306] -> w272
              disable-tunnel: w274 -> [w281 _]
              disable-tunnel: w275 -> [w280 _]
              frame condition #0 (active) {
                n103 = case shown="\"Open\"" w280 {
                  tunnel: w283 -> [w287 w300]
                  tunnel: [w289 w301] -> w282
                  tunnel: w281 -> [w288 w298]
                  frame "Open" {
                    # "Open FP if not open or invalid"
                    n104 = property class="VI"(reference=w288, error in=w287) -> (reference out=w285:refnum<vi>, error out=w286:errorcluster, "FP.State"=w284:T6)
                    n105 = case shown="Default" w284 {
                      tunnel: [w292 w295] -> w289
                      tunnel: w286 -> [w291 w295]
                      tunnel: w285 -> [w290 _]
                      frame Default {
                        n106 = invoke class="VI" method="FP.Open"(reference=w290, error in=w291, "Activate"=TRUE, "State"=T6."Standard") -> (error out=w292:errorcluster)  [unwired: 1 in, 4 out]
                      }
                      frame "Invalid", "Standard" {
                      }
                    }
                  }
                  frame "Close", Default {
                    # "Close FP is not Closed or Invalid"
                    n107 = property class="VI"(reference=w298, error in=w300) -> (reference out=w297:refnum<vi>, error out=w299:errorcluster, "FP.State"=w296:T6)
                    n108 = case shown="Default" w296 {
                      tunnel: [w302 w305] -> w301
                      tunnel: w299 -> [w302 w304]
                      tunnel: w297 -> [_ w303]
                      frame "Invalid", "Closed" {
                      }
                      frame Default {
                        n109 = invoke class="VI" method="FP.Close"(reference=w303, error in=w304) -> (error out=w305:errorcluster)  [unwired: 1 in, 2 out]
                      }
                    }
                  }
                }
              }
              frame condition #1 {
              }
            }
            n110 = call <vilib>:"Add State(s) to Queue__jki_lib_state_machine.vi"("State(s) in (\"\")"=w279) -> ("States Out"=w278:string)  [unwired: 14 in]
          }
          frame "---------- Macro ----------" {
            # "Do not put any code in this frame.\n(It is a separator no-op. You can make a copy of this frame to create a new Macro frame)"
            n111 = call <vilib>:"Add State(s) to Queue__jki_lib_state_machine.vi"("State(s) in (\"\")"=w311) -> ("States Out"=w310:string)  [unwired: 14 in]
          }
          frame "Macro: Initialize" {
            w315 = "UI: Initialize\n//UI: Front Panel State >> Open\n\n//Test: Start SMO Dependency //Only for development purpose."  # UI: Initialize //UI: Front Panel State >> Open  //Test: Start SMO Dependency //Only for development purpose.
            # "Initialization Macro\n(This is called once, when the VI starts)"
            n112 = call <vilib>:"Add State(s) to Queue__jki_lib_state_machine.vi"("State(s) in Front (\"\")"="Data: Initialize\nInitialize Core Data\nEvents: Register", "State(s) in (\"\")"="Process: Sync", "State(s) at Back (\"\")"=w315) -> ("States Out"=w314:string)  [unwired: 12 in]
            n113 = call <vilib>:"Add State(s) to Queue__jki_lib_state_machine.vi"("State(s) in Front (\"\")"=w314, "State(s) in (\"\")"=w320) -> ("States Out"=w319:string)  [unwired: 13 in]
          }
          frame "Macro: Start Req Analysis" {
            n114 = call <vilib>:"Add State(s) to Queue__jki_lib_state_machine.vi"("State(s) in Front (\"\")"="UI: Update\nSReTT: Timer >> Start\nFile IO: Setup\nFile IO: Get New Requirement File\nSReTT: Postprocess\nSReTT: Timer >> Stop\nUI: Update" ("State(s) in Front (\"\")"), "State(s) in (\"\")"=w326) -> ("States Out"=w325:string)  [unwired: 13 in]
          }
          frame "Macro: Exit" {
            # "Exit Macro\n(This is called once, when the VI exits)"
            n115 = Unbundle By Name(w328) -> ("Core.Close Panel on Exit?"=w334:bool)
            n116 = Select(t="UI: Front Panel State >> Close", s=w334, f="") -> (s? t:f=w331:string)
            n117 = call <vilib>:"Add State(s) to Queue__jki_lib_state_machine.vi"("State(s) in (\"\")"=w331, "State(s) at Back (\"\")"="Data: Cleanup\nEvents: Unregister\nProcess: Sync\nExit") -> ("States Out"=w330:string)  [unwired: 13 in]
            n118 = call <vilib>:"Add State(s) to Queue__jki_lib_state_machine.vi"("State(s) in Front (\"\")"=w330, "State(s) in (\"\")"=w337) -> ("States Out"=w336:string)  [unwired: 13 in]
          }
          frame "---------- Process ----------" {
            # "Template Separator\n(You can make a copy of, or modify, this frame)"
            n119 = call <vilib>:"Add State(s) to Queue__jki_lib_state_machine.vi"("State(s) in (\"\")"=w342) -> ("States Out"=w341:string)  [unwired: 14 in]
          }
          frame "Process: Sync" {
            n120 = Unbundle By Name(w350) -> ("Self Ref"=w346:refnum<class "Analyzer.lvclass">)
            n121 = call <vilib>:"WaitOnProcessSync.vi"("error in (no error)"=w345, "SMO"=w346) -> ("error out"=w344:errorcluster, "Don't run?"=w349:bool)  [unwired: 7 in, 1 out]
            n122 = Select(t="Data: Cleanup\nEvents: Unregister\nExit", s=w349, f="") -> (s? t:f=w343:string)
            n123 = call <vilib>:"Add State(s) to Queue__jki_lib_state_machine.vi"("State(s) in Front (\"\")"=w343, "State(s) in (\"\")"=w353) -> ("States Out"=w352:string)  [unwired: 13 in]
          }
          frame "Test: Start SMO Dependency" {
            # ">> Returns the instance of \"Dummy\"\nand ignores the other levels dependencies"
            n124 = Unbundle By Name(w362) -> ("Self Ref"=w361:refnum<class "Analyzer.lvclass">)
            n125 = call <vilib>:"LaunchDependency.vi"("error in (no error)"=w357, "Dependency Name"="Dummy", "Dependency Type"=refnum<class "SMO.lvclass"> refnum ("SMO.lvclass"), "SMO in"=w361) -> ("error out"=w360:errorcluster, "SMO out"=w354:refnum<class "Analyzer.lvclass">)  [unwired: 4 in, 2 out]
            n126 = call <vilib>:"ListThisLevelDependencies.vi"("SMO in"=w354) -> ("[My Dependencies]"=w356:refnum<class "SMO.lvclass">[])  [unwired: 8 in, 2 out]
            n127 = Index Array(array=w356) -> (element=w355:refnum<class "SMO.lvclass">)  [unwired: 1 in]
            n128 = call <vilib>:"Get Name.vi"("SMO"=w355) -> ()  [unwired: 6 in, 5 out]
            n129 = call <vilib>:"Add State(s) to Queue__jki_lib_state_machine.vi"("State(s) in (\"\")"=w365) -> ("States Out"=w364:string)  [unwired: 14 in]
          }
          frame "---------- Events ----------" {
            # "Template Separator\n(You can make a copy of, or modify, this frame)"
            n130 = call <vilib>:"Add State(s) to Queue__jki_lib_state_machine.vi"("State(s) in (\"\")"=w370) -> ("States Out"=w369:string)  [unwired: 14 in]
          }
          frame "Events: Register" {
            n131 = Unbundle By Name(w383) -> ("Self Ref"=w379:refnum<class "Analyzer.lvclass">)
            n132 = call <vilib>:"GetProtectedEvents.vi"("error in (no error)"=w375, "SMO"=w379) -> ("error out"=w376:errorcluster, "SMO Protected Events"=w382:T11, "SMO out"=w377:refnum<class "Analyzer.lvclass">)  [unwired: 7 in]
            n133 = call "Analyzer.GetPublicEvents.vi"("error in (no error)"=w376, "Analyzer"=w377) -> ("error out"=w372:errorcluster, "SMO.Analyzer Public Events"=w378:T12, "Analyzer out"=w374:refnum<class "Analyzer.lvclass">)  [unwired: 7 in]
            n134 = call "Analyzer.GetPrivateEvents.vi"("error in (no error)"=w372, "Analyzer"=w374) -> ("error out"=w371:errorcluster, "Analyzer Private Events"=w373:T13)  [unwired: 7 in, 1 out]
            n135 = register-events(error in=w371, w382, w378, w373) -> (reference out=w380:refnum<event-registration>, error out=w381:errorcluster)  [unwired: 1 in]
            n136 = call <vilib>:"Add State(s) to Queue__jki_lib_state_machine.vi"("State(s) in (\"\")"=w385) -> ("States Out"=w384:string)  [unwired: 14 in]
          }
          frame "Events: Unregister" {
            # "Your code here.\n(You can make a copy of, or modify, this frame)"
            n137 = Unregister For Events(event registration refnum=w388, error in=w387) -> (error out=w386:errorcluster)
            n138 = call <vilib>:"Clear Errors.vi"("error in (no error)"=w386) -> ()  [unwired: 5 in, 2 out]
            n139 = call <vilib>:"Add State(s) to Queue__jki_lib_state_machine.vi"("State(s) in (\"\")"=w391) -> ("States Out"=w390:string)  [unwired: 14 in]
          }
          frame "---------- File IO ----------" {
            # "MsgAction Separator\n(You can make a copy of, or modify, this frame)"
          }
          frame "File IO: Setup" {
            n140 = Unbundle By Name(w405) -> ("Settings.Source Code Directory"=w397:path, "Settings.Requirements Directory"=w404:path)
            n141 = call "Analyzer.RequirementFileNameObtainer.vi"("CSV Directory"=w404, "Operation"=enum16{"Reset", "Get"}."Reset", "error in"=w406) -> ("error out"=w398:errorcluster)  [unwired: 10 in, 2 out]
            n142 = call "Analyzer.CodeFileNameObtainer.vi"("Code Directory"=w397, "Operation"=enum16{"Reset", "Get"}."Reset", "error in"=w398) -> ("error out"=w396:errorcluster)  [unwired: 10 in, 2 out]
            n143 = call "Analyzer.CodeFileNameObtainer.vi"("Code Directory"=w397, "Operation"=enum16{"Reset", "Get"}."Get", "error in"=w396) -> ("File Path"=w400:path, "error out"=w402:errorcluster)  [unwired: 10 in, 1 out]
            n144 = Bundle By Name(cluster=w405, "Settings.Source Code File"=w400) -> (w403:T9)
          }
          frame "File IO: Get New Requirement File" {
            n145 = call "Analyzer.GetRequirement_FGV.vi"("Operation"=enum16{"Reset", "Get"}."Reset", "error in"=w415) -> ("error out"=w410:errorcluster)  [unwired: 7 in, 2 out]
            n146 = Unbundle By Name(w428) -> ("S Word Ctrl"=w412:bool, "Requirements"=w413:string[], "Single Word"=w414:bool, "Settings.Requirements Directory"=w426:path)
            n147 = case shown="False" w414 {
              tunnel: [w433 w437] -> w427
              tunnel: w426 -> [w430 _]
              tunnel: [w432 w436] -> w425
              tunnel: [w431 w435] -> w422
              tunnel: w410 -> [w434 w437]
              tunnel: w413 -> [_ w436]
              tunnel: w412 -> [_ w435]
              frame False {
                n148 = call "Analyzer.CSVFileNameParser.vi"("error in (no error)"=w434, "Requirements Definition (.csv)"=w430) -> ("error out"=w433:errorcluster, "No more elements"=w431:bool, "Requirements"=w432:string[])  [unwired: 7 in]
              }
              frame True {
              }
            }
            n149 = Bundle By Name(cluster=w428, "S Word Ctrl"=TRUE, "Requirements"=w425, "Req Files Done"=w422) -> (w421:T9)
            n150 = Unbundle By Name(w421) -> ("Req Files Done"=w420:bool)
            n151 = Select(t="", s=w420, f="SReTT: Get New Requirement") -> (s? t:f=w418:string)
            n152 = call <vilib>:"Add State(s) to Queue__jki_lib_state_machine.vi"("State(s) in Front (\"\")"=w418, "State(s) in (\"\")"=w423) -> ("States Out"=w424:string)  [unwired: 13 in]
          }
          frame "File IO: Reset Req List" {
            # "MsgAction Separator\n(You can make a copy of, or modify, this frame)"
            n153 = call "Analyzer.GetRequirement_FGV.vi"("Operation"=enum16{"Reset", "Get"}."Reset") -> ()  [unwired: 8 in, 3 out]
          }
          frame "File IO: Get New Code File" {
            n154 = Unbundle By Name(w456) -> ("Settings.Source Code Directory"=w445:path)
            n155 = call "Analyzer.CodeFileNameObtainer.vi"("Code Directory"=w445, "Operation"=enum16{"Reset", "Get"}."Get", "error in"=w457) -> ("File Path"=w453:path, "End of List"=w454:bool, "error out"=w455:errorcluster)  [unwired: 10 in]
            n156 = Bundle By Name(cluster=w456, "Settings.Source Code File"=w453, "Code Files Done"=w454) -> (w444:T9)
            n157 = Unbundle By Name(w444) -> ("Code Files Done"=w446:bool)
            n158 = case shown="True" w446 {
              tunnel: [_ w465] -> _
              tunnel: w445 -> [_ w460]
              tunnel: w444 -> [w459 w463]
              tunnel: [w459 w462] -> w443
              frame False {
              }
              frame True {
                n159 = call "Analyzer.CodeFileNameObtainer.vi"("Code Directory"=w460, "Operation"=enum16{"Reset", "Get"}."Reset") -> ("error out"=w466:errorcluster)  [unwired: 11 in, 2 out]
                n160 = call "Analyzer.CodeFileNameObtainer.vi"("Code Directory"=w460, "Operation"=enum16{"Reset", "Get"}."Get", "error in"=w466) -> ("File Path"=w461:path, "error out"=w465:errorcluster)  [unwired: 10 in, 1 out]
                n161 = Bundle By Name(cluster=w463, "Settings.Source Code File"=w461) -> (w462:T9)
              }
            }
            n162 = Select(t="File IO: Get New Requirement File", s=w446, f="SReTT: Get New Requirement") -> (s? t:f=w447:string)
            n163 = call <vilib>:"Add State(s) to Queue__jki_lib_state_machine.vi"("State(s) in Front (\"\")"=w447, "State(s) in (\"\")"=w450) -> ("States Out"=w451:string)  [unwired: 13 in]
          }
          frame "---------- SReTT ----------" {
            # "MsgAction Separator\n(You can make a copy of, or modify, this frame)"
          }
          frame "SReTT: Postprocess" {
            n164 = call <vilib>:"Add State(s) to Queue__jki_lib_state_machine.vi"("State(s) in (\"\")"=w473) -> ("States Out"=w474:string)  [unwired: 14 in]
          }
          frame "SReTT: Get New Requirement" {
            n165 = Unbundle By Name(w484) -> ("Requirements"=w483:string[])
            n166 = call "Analyzer.GetRequirement_FGV.vi"("Operation"=enum16{"Reset", "Get"}."Get", "List of Words"=w483) -> ("Word for search"=w480:string)  [unwired: 7 in, 2 out]
            n167 = Empty String/Path?(string/path=w480) -> (empty?=w478:bool)
            n168 = case shown="True" w478 {
              tunnel: w484 -> [w491 w494]
              tunnel: w480 -> [w490 _]
              tunnel: [w489 w494] -> w479
              tunnel: ["SReTT: Main" "File IO: Get New Code File"] -> w477
              frame False {
                n169 = Bundle By Name(cluster=w491, "Requirement to Look"=w490) -> (w489:T9)
              }
              frame True {
                n170 = call "Analyzer.GetRequirement_FGV.vi"("Operation"=enum16{"Reset", "Get"}."Reset") -> ()  [unwired: 8 in, 3 out]
              }
            }
            n171 = call <vilib>:"Add State(s) to Queue__jki_lib_state_machine.vi"("State(s) in Front (\"\")"=w477, "State(s) in (\"\")"=w481) -> ("States Out"=w482:string)  [unwired: 13 in]
          }
          frame "SReTT: Main" {
            w514 = "search_word_in_file"  # function name
            n172 = Unbundle By Name(w511) -> ("Python.Ref"=w512:refnum<k35>, "Python.SReTT_script"=w513:path, "Settings.Source Code File"=w503:path, "Requirement to Look"=w502:string, "Table"=w497:string[][])
            n173 = Path To String(path=w503) -> (string=w504:string)
            n174 = node(w512, w513, w514, w506, string[] [], w504, w502) -> (w509:refnum<k35>, w505:errorcluster, w499:string[])  [unwired: 2 in, 2 out]
            n175 = Build Array (concatenate)(w497, w499) -> (w496:string[][])
            n176 = Empty Array?(array=w499) -> (empty?=w498:bool)
            n177 = Select(t=w497, s=w498, f=w496) -> (s? t:f=w495:string[][])
            n178 = Bundle By Name(cluster=w511, "Python.Ref"=w509, "Table"=w495) -> (w510:T9)
            n179 = call <vilib>:"Add State(s) to Queue__jki_lib_state_machine.vi"("State(s) in Front (\"\")"="SReTT: Get New Requirement" ("State(s) in Front (\"\")"), "State(s) in (\"\")"=w507) -> ("States Out"=w508:string)  [unwired: 13 in]
          }
          frame "SReTT: Timer" {
            n180 = Enqueue Element(queue=w519, element=w516, error in (no error)=w518) -> (error out=w517:errorcluster)  [unwired: 1 in, 2 out]
          }
          frame "---------- Report ----------" {
            # "MsgAction Separator\n(You can make a copy of, or modify, this frame)"
          }
          frame "Report: Main" {
            n181 = Unbundle By Name(w542) -> ("Settings.Report Generation Save Path"=w541:path, "Table"=w535:string[][])
            n182 = Get Date/Time In Seconds() -> (seconds since 1Jan1904=w539:timestamp)
            n183 = Format Date/Time String(time format string (%c)="Report_%d%m%y_%H%M%S.csv", seconds (now)=w539) -> (date/time string=w537:string)  [unwired: 1 in]
            n184 = Insert Into Array(array=w535, index (row)=0, new element=string[] ["Requirement ID", "Found?", "File Path", "Line Number", "Code"] ("new element/subarray")) -> (w534:string[][])  [unwired: 1 in]
            n185 = Build Path(base path=w541, name or relative path=w537) -> (appended path=w528:path)
            n186 = Path To String(path=w528) -> (string=w527:string)
            n187 = call-poly <vilib>:"Write Delimited Spreadsheet.vi"("file path (dialog if empty)"=w528, "2D data"=w534, "error in (no error)"=w540, "delimiter (\\t)"="," ("delimiter (\\t)")) -> ("error out"=w531:errorcluster)  [unwired: 10 in, 1 out]
            n188 = Concatenate Strings("Report Created Succesfully.\nLocation: " ("time format string (%c)"), w527) -> (w529:string)
            n189 = case shown="No Error" w531 {
              tunnel: w529 -> [w545 _]
              frame No Error {
                n190 = One Button Dialog(message=w545) -> ()  [unwired: 1 in, 1 out]
              }
              frame Error {
              }
            }
          }
        }
      }
      n191 = call "Analyzer.Timer.vi"("error in (no error)"=w12, "Queue"=w13, "Analyzer in"=w14) -> ()  [unwired: 8 in, 1 out]
    }
    frame Error {
    }
  }
  n192 = call-parent "Process.vi"("error in"=w11, "SMO"=w1) -> ("error out"=w10:errorcluster, "SMO out"=→"Analyzer out":refnum<class "Analyzer.lvclass">)  [unwired: 8 in]
  n193 = Merge Errors(w10, w9) -> (→"error out":errorcluster)
